vi "find device.vi"(8 "error in (no error)":errorcluster, 11 "USB IO in":refnum<class "USB IO.lvclass">) -> (0 "error out":errorcluster, 3 "USB IO out":refnum<class "USB IO.lvclass">)   [LabVIEW 2025, in "USB IO.lvlib" / "USB IO.lvclass"]
uses:
  USB IO.lvclass
  USB IO.lvclass/USB IO.ctl
  <resource>/objmgr/daqmx.rc
panel:
  out "AI.PhysicalChans":tag[](array[tag])
  out "DO.Ports":tag[](array[tag])
  out "DO.Lines":tag[](array[tag])
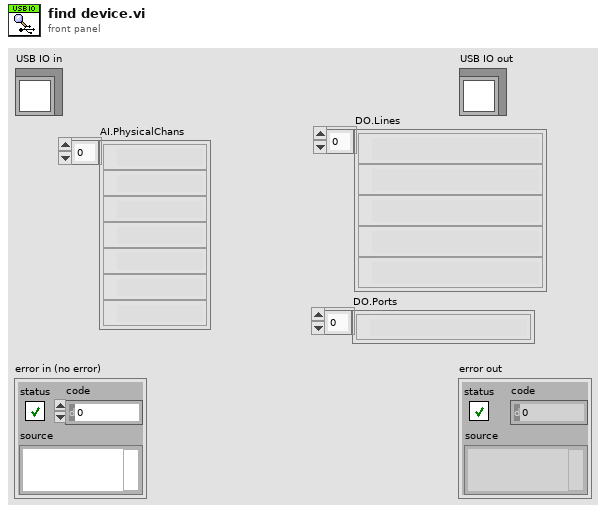
[diagram p1: front panel]
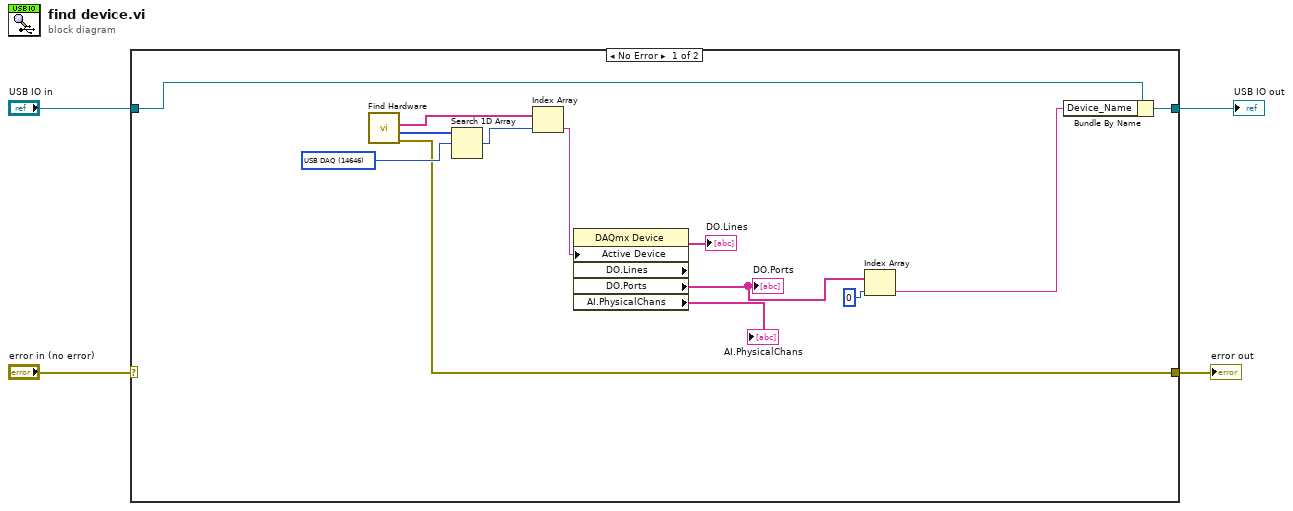
[diagram p0: block diagram]
diagram:
  n1 = case shown="No Error" "error in (no error)" {
    selector: "error in (no error)" -> [_ w19]
    tunnel: [w11 w19] -> w3
    tunnel: [w13 w18] -> w1
    tunnel: "USB IO in" -> [w12 w18]
    frame No Error {
      w16 = 14646 items=["M Series DAQ"=14643, "X Series DAQ"=15858, "E Series DAQ"=14642, "S Series DAQ"=14644, "B Series DAQ"=14662, "SC Series DAQ"=14645, "USB DAQ"=14646, "AO Series"=14647, "Digital I/O"=14648, "TIO Series"=14661, "Dynamic Signal Acquisition"=14649, "Switches"=14650, "CompactDAQ Chassis"=14658, "CompactRIO Chassis"=16144, "C Series Module"=14659, "SCXI Module"=14660, "SCC Connector Block"=14704, "SCC Module"=14705, "NI ELVIS"=14755, "Network DAQ"=14829, "SC Express"=15886, "FieldDAQ"=16151, "TestScale Chassis"=16180, "TestScale Module"=16181, "mioDAQ"=16182, "Unknown"=12588] ("ProductCategory")
      n2 = call "Find Hardware.vi"() -> ("error out"=w11:errorcluster, "Product Category"=w17:i32[], "DevNames"=w15:tag[])  [unwired: 8 in, 1 out]
      n3 = Search 1D Array(1D array=w17, element=w16) -> (index of element=w14:i32)  [unwired: 1 in]
      n4 = Index Array(array=w15, index=w14) -> (element=w10:tag)
      n5 = property class="DAQmx Device"("Active Device"=w10) -> ("DO.Lines"=→"DO.Lines":tag[], "DO.Ports"=w8:tag[], "AI.PhysicalChans"=→"AI.PhysicalChans":tag[])  [unwired: 2 in, 2 out]
      "DO.Ports" <- w8
      n6 = Index Array(array=w8, index=0) -> (element=w6:tag)
      n7 = Bundle By Name(cluster=w12, "Device_Name"=w6) -> (w13:refnum<class "USB IO.lvclass">)
    }
    frame Error {
    }
  }
  "error out" <- w3
  "USB IO out" <- w1
